vi "ActionVIOnCompile.vi"(8 "error in (no error)":errorcluster, 11 "Device Item Ref in":T1 format="%.0x") -> (0 "error out":errorcluster)   [LabVIEW 2015, in "J1939 Addon System Explorer.lvlib"]
uses:
  J1939 Addon System Explorer.lvlib
  <vilib>/NI Veristand/Custom Device API/Custom Device Item Ref.ctl
  Shared/Types/Compile Addon Settings.ctl
  Shared/Types/XNET Settings.ctl
  Shared/Types/SysDef FPGA Settings.ctl
  Shared/Types/Compiled.Node Settings.ctl
  Shared/Types/Compiled Monitor Tool Settings.ctl
  Shared/Types/Monitor Settings.ctl
  Shared/Types/Device Settings.ctl
  Shared/Types/Incoming Settings.ctl
  Shared/Types/Frame Settings.ctl
  Shared/Types/Outgoing Event Trigger Types.ctl
  <vilib>/NI Veristand/Custom Device API/Block Data Reference.ctl
  <vilib>/NI Veristand/Custom Device API/Data Reference.ctl
  Shared/Types/Outgoing Settings.ctl
  Shared/Types/Complied Simulated Device Settings.ctl
  Shared/Types/Compiled Simulated Settings.ctl
  Shared/SubVIs/Constants.vi
  <vilib>/NI Veristand/Custom Device API/Set Item Property (Variant).vi
  Shared/J1939 Addon Shared.lvlib
  <vilib>/NI VeriStand/Custom Device API/Custom Device API.lvlib
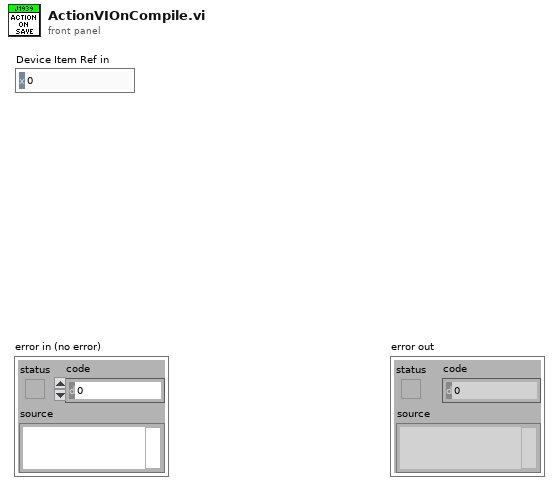
[diagram p1: front panel]
types:
  T1 = typedef "Custom Device API.lvlib/Custom Device Item Ref.ctl" = u64
  T2 = typedef "J1939 Addon Shared.lvlib/Compile Addon Settings.ctl" = cluster{"XNET":T3, "Bitfile":T4, "Nodes":T5, "Name":string}
  T3 = typedef "J1939 Addon Shared.lvlib/XNET Settings.ctl" = cluster{"Database":refnum<k21>, "Cluster":refnum<k21>, "Port":string, "Baud rate [Bd]":u32, "Termination":u32, "Incoming Decimation":u32, "Outgoing Decimation":u32}
  T4 = typedef "J1939 Addon Shared.lvlib/SysDef FPGA Settings.ctl" = cluster{"RT Path":path, "RIO Device":u16, "Enable":bool}
  T5 = typedef "J1939 Addon Shared.lvlib/Compiled.Node Settings.ctl" = cluster{"Monitor":T6, "Sim":T15[]}
  T6 = typedef "J1939 Addon Shared.lvlib/Compiled Monitor Tool Settings.ctl" = cluster{"Network":T7, "Data":T8}
  T7 = typedef "J1939 Addon Shared.lvlib/Monitor Settings.ctl" = cluster{"Address":u8, "Name":u64}
  T8 = typedef "J1939 Addon Shared.lvlib/Device Settings.ctl" = cluster{"Incoming":T9, "Outgoing":T14}
  T9 = typedef "J1939 Addon Shared.lvlib/Incoming Settings.ctl" = cluster{"Signals":string[], "Frames":T10[], "Data.Refs":T12[], "Data.Values":dbl[], "Timing.Use":bool, "Timing.Refs":T12[], "Timing.Values":dbl[], "Timing.Index":i32[]}
  T10 = typedef "J1939 Addon Shared.lvlib/Frame Settings.ctl" = cluster{"Signals":string[], "Channel Array Position":cluster{"Offset":u32, "Length":u32}, "PGN":u32, "Cyclic?":bool, "Disable?":bool, "Disable.Index":i32, "Trigger":T11, "Trigger.Index":i32}
  T11 = typedef "J1939 Addon Shared.lvlib/Outgoing Event Trigger Types.ctl" = enum16{"Channel value change", "Trigger channel (not zero)", "Channel value change or trigger channel (not zero)", "Trigger channel (any value change)", "Channel value change or trigger channel (any value change)"}
  T12 = typedef "Custom Device API.lvlib/Block Data Reference.ctl" = cluster{"Data Reference":T13, "Offset":u64, "Length":u64}
  T13 = typedef "Custom Device API.lvlib/Data Reference.ctl" = i32
  T14 = typedef "J1939 Addon Shared.lvlib/Outgoing Settings.ctl" = cluster{"Frames":T10[], "Data.Refs":T12[], "Data.Values":dbl[], "Disable.Refs":T12[], "Disable.Values":dbl[], "Trigger.Refs":T12[], "Trigger.Values":dbl[]}
  T15 = typedef "J1939 Addon Shared.lvlib/Complied Simulated Device Settings.ctl" = cluster{"Network":T7, "Data":T8, "DTCs":T16}
  T16 = typedef "J1939 Addon Shared.lvlib/Compiled Simulated Settings.ctl" = cluster{"DM1.Ref":T12[], "DM1.Value":dbl[], "DM1.Enable.Ref":T12[], "DM1.Enable.Value":dbl[], "DM2.Ref":T12[], "DM2.Value":dbl[], "DM2.Enable.Ref":T12[], "DM2.Enable.Value":dbl[]}
  T17 = typedef "Custom Device API.lvlib/Custom Device Item Info.ctl" = cluster{"Name":string, "Is Channel":bool, "GUID":string, "Is Waveform":bool}
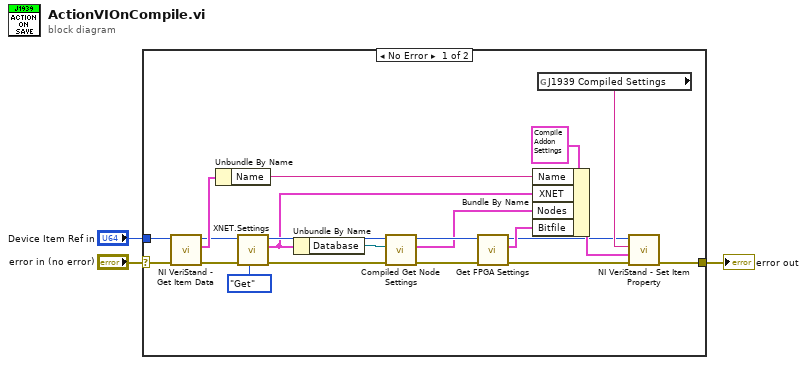
[diagram p0: block diagram]
diagram:
  n1 = case shown="No Error" "error in (no error)" {
    selector: "error in (no error)" -> [w10 w25]
    tunnel: [w20 w25] -> w2
    tunnel: "Device Item Ref in" -> [w11 _]
    frame No Error {
      n2 = call <vilib>:"NI VeriStand - Get Item Data.vi"("error in (no error)"=w10, "Item Ref in"=w11) -> ("error out"=w5:errorcluster, "Item Info"=w12:T17, "Item Ref out"=w4:T1)  [unwired: 6 in, 1 out]
      n3 = Unbundle By Name(w12) -> ("Name"=w9:string)
      n4 = call "XNET.Settings.vi"("Action"=enum8{"Get", "Set"}."Get", "error in (no error)"=w5, "Parent Ref in"=w4) -> ("error out"=w6:errorcluster, "J1939 XNET Settings"=w7:T3, "Item Ref out"=w24:T1)  [unwired: 6 in]
      n5 = Unbundle By Name(w7) -> ("Database"=w16:refnum<k21>)
      n6 = call "Compiled Get Node Settings.vi"("error in"=w6, "database in"=w16, "Addon Ref"=w24) -> ("error out"=w15:errorcluster, "J1939 Data Settings"=w13:T5, "Addon Ref out"=w14:T1)  [unwired: 6 in]
      n7 = call "Get FPGA Settings.vi"("error in (no error)"=w15, "Item Ref in"=w14) -> ("error out"=w21:errorcluster, "FPGA Bitfile Settings"=w22:T4, "Item Ref out"=w17:T1)  [unwired: 7 in]
      n8 = Bundle By Name(cluster=T2 {"XNET"={"Database"="", "Cluster"="", "Port"="", "Baud rate [Bd]"=0, "Termination"=0, "Incoming Decimation"=0, "Outgoing Decimation"=0}, "Bitfile"={"RT Path"=path "", "RIO Device"=0, "Enable"=FALSE}, "Nodes"={"Monitor"={"Network"={"Address"=0, "Name"=0}, "Data"={"Incoming"={"Signals"=[], "Frames"=[], "Data.Refs"=[], "Data.Values"=[], "Timing.Use"=FALSE, "Timing.Refs"=[], "Timing.Values"=[], "Timing.Index"=[]}, "Outgoing"={"Frames"=[], "Data.Refs"=[], "Data.Values"=[], "Disable.Refs"=[], "Disable.Values"=[], "Trigger.Refs"=[], "Trigger.Values"=[]}}}, "Sim"=[]}, "Name"=""}, "Name"=w9, "XNET"=w7, "Nodes"=w13, "Bitfile"=w22) -> (w19:T2)
      n9 = global read "Constants.vi" "J1939 Compiled Settings"() -> (w18:string)
      n10 = call-poly <vilib>:"NI VeriStand - Set Item Property.vi"("error in (no error)"=w21, "Value"=w19, "Property Name"=w18, "Item Ref in"=w17) -> ("error out"=w20:errorcluster)  [unwired: 5 in, 2 out]
    }
    frame Error {
    }
  }
  "error out" <- w2
